vi "Write Key.vi"(6 "section":string, 7 "data type":T1, 8 "error in (no error)":errorcluster, 9 "key":variant, 10 "name":string, 11 "Configuration.lvclass in":refnum<class "Configuration.lvclass">) -> (0 "error out":errorcluster, 3 "Configuration.lvclass out":refnum<class "Configuration.lvclass">)   [LabVIEW 2011, in "Configuration.lvclass"]
uses:
  Configuration.lvclass
  Key Data Type.ctl
  Configuration.lvclass/Configuration.ctl
  <vilib>/Utility/config.llb/Write Key (Boolean).vi
  <vilib>/Utility/config.llb/Write Key (U32).vi
  <vilib>/Utility/config.llb/Write Key (I32).vi
  <vilib>/Utility/config.llb/Write Key (Double).vi
  <vilib>/Utility/config.llb/Write Key (String).vi
  <vilib>/Utility/config.llb/Write Key (Path).vi
  <vilib>/Utility/config.llb/NI_LVConfig.lvlib
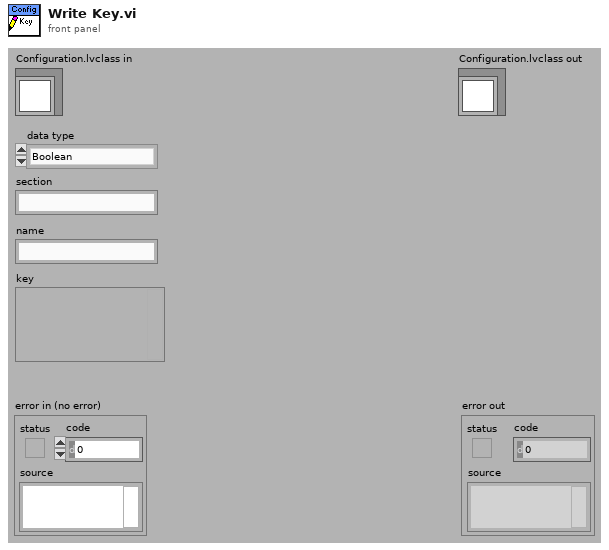
[diagram p1: front panel]
types:
  T1 = typedef "Configuration.lvclass/Key Data Type.ctl" = enum16{"Boolean", "U32", "I32", "Double", "String", "DAQmx Channel", "Path"}
  T2 = typedef "NI_LVConfig.lvlib/Config Data RefNum.ctl" = refnum<k1>
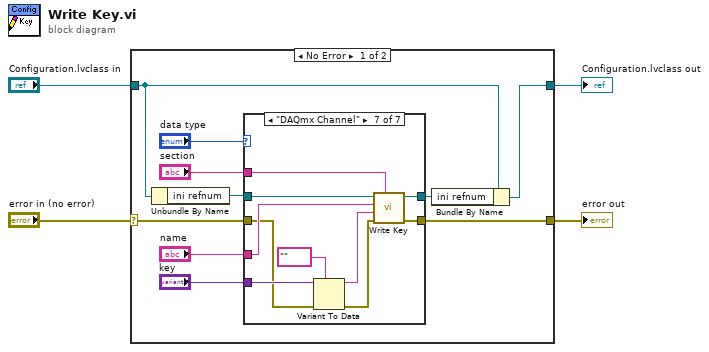
[diagram p0: block diagram]
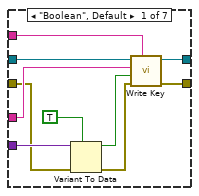
[diagram p2: hidden frame]
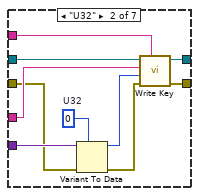
[diagram p3: hidden frame]
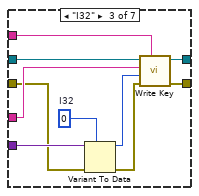
[diagram p4: hidden frame]
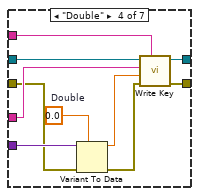
[diagram p5: hidden frame]
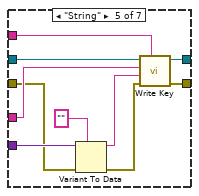
[diagram p6: hidden frame]
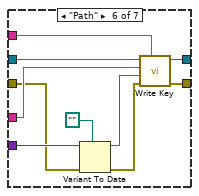
[diagram p7: hidden frame]
diagram:
  n1 = case shown="No Error" "error in (no error)" {
    selector: "error in (no error)" -> [w9 w85]
    tunnel: [w8 w85] -> w3
    tunnel: [w5 w86] -> w1
    tunnel: "Configuration.lvclass in" -> [w7 w86]
    frame No Error {
      n2 = Unbundle By Name(w7) -> ("ini refnum"=w13:T2)
      n3 = case shown="\"DAQmx Channel\"" "data type" {
        tunnel: "section" -> [w24 w34 w44 w54 w64 w74 w84]
        tunnel: w13 -> [w23 w33 w43 w53 w63 w73 w83]
        tunnel: [w21 w31 w41 w51 w61 w71 w81] -> w6
        tunnel: "name" -> [w22 w32 w42 w52 w62 w72 w82]
        tunnel: [w17 w28 w38 w47 w57 w67 w78] -> w8
        tunnel: "key" -> [w20 w30 w40 w50 w60 w70 w80]
        tunnel: w9 -> [w16 w26 w36 w46 w56 w66 w76]
        frame "Boolean", Default {
          n4 = Variant To Data(error in=w16, type=TRUE, Variant=w20) -> (data=w18:bool, error out=w15:errorcluster)
          n5 = call-poly <vilib>:"Write Key.vi"("section"=w24, "error in (no error)"=w15, "value"=w18, "key"=w22, "refnum"=w23) -> ("error out"=w17:errorcluster, "refnum out"=w21:T2)  [unwired: 4 in, 1 out]
        }
        frame "U32" {
          w27 = u32 0  # U32
          n6 = Variant To Data(error in=w26, type=w27, Variant=w30) -> (data=w29:u32, error out=w25:errorcluster)
          n7 = call-poly <vilib>:"Write Key.vi"("section"=w34, "error in (no error)"=w25, "value"=w29, "key"=w32, "refnum"=w33) -> ("error out"=w28:errorcluster, "refnum out"=w31:T2)  [unwired: 4 in, 1 out]
        }
        frame "I32" {
          w37 = 0  # I32
          n8 = Variant To Data(error in=w36, type=w37, Variant=w40) -> (data=w39:i32, error out=w35:errorcluster)
          n9 = call-poly <vilib>:"Write Key.vi"("section"=w44, "error in (no error)"=w35, "value"=w39, "key"=w42, "refnum"=w43) -> ("error out"=w38:errorcluster, "refnum out"=w41:T2)  [unwired: 4 in, 1 out]
        }
        frame "Double" {
          w48 = 0.0  # Double
          n10 = Variant To Data(error in=w46, type=w48, Variant=w50) -> (data=w49:dbl, error out=w45:errorcluster)
          n11 = call-poly <vilib>:"Write Key.vi"("section"=w54, "error in (no error)"=w45, "value"=w49, "key"=w52, "refnum"=w53) -> ("error out"=w47:errorcluster, "refnum out"=w51:T2)  [unwired: 4 in, 1 out]
        }
        frame "String" {
          n12 = Variant To Data(error in=w56, type="", Variant=w60) -> (data=w59:string, error out=w55:errorcluster)
          n13 = call-poly <vilib>:"Write Key.vi"("section"=w64, "error in (no error)"=w55, "value"=w59, "key"=w62, "refnum"=w63) -> ("error out"=w57:errorcluster, "refnum out"=w61:T2)  [unwired: 4 in, 1 out]
        }
        frame "Path" {
          n14 = Variant To Data(error in=w66, type=path "", Variant=w70) -> (data=w69:path, error out=w65:errorcluster)
          n15 = call-poly <vilib>:"Write Key.vi"("section"=w74, "error in (no error)"=w65, "value"=w69, "key"=w72, "refnum"=w73) -> ("error out"=w67:errorcluster, "refnum out"=w71:T2)  [unwired: 4 in, 1 out]
        }
        frame "DAQmx Channel" {
          n16 = Variant To Data(error in=w76, type=tag "" ("PID DAQmx Channels.S2"), Variant=w80) -> (data=w79:tag, error out=w75:errorcluster)
          n17 = call-poly <vilib>:"Write Key.vi"("section"=w84, "error in (no error)"=w75, "value"=w79, "key"=w82, "refnum"=w83) -> ("error out"=w78:errorcluster, "refnum out"=w81:T2)  [unwired: 4 in, 1 out]
        }
      }
      n18 = Bundle By Name(cluster=w7, "ini refnum"=w6) -> (w5:refnum<class "Configuration.lvclass">)
    }
    frame Error {
    }
  }
  "error out" <- w3
  "Configuration.lvclass out" <- w1
